vi "Run_6_of_6_Tests.vi"() -> ()   [LabVIEW 2019]
uses:
  <vilib>/Rock Robotics/WPI/ThirdParty/JAS_Junk/TrajLib/Trajectory_Library.lvlib
panel:
  out "Vector":bool
  out "Lead Lag":bool
  out "Pose3d":bool
  out "Transform3d":bool
  out "Rotation3d":bool
  out "Translation3d":bool
  out "Twist3d":bool
  out "Function Generator \nMatrix":bool
  out "LTV Unicycle \nController":bool
  out "LTV Diff Drive \nController":bool
  out "Time Interpolatable Rotation":bool
  out "Time Interpolatable Double":bool
  out "Time Interpolatable Boolean":bool
  out "Time Interpolatable Pose":bool
  out "Implicit Model Follower":bool
  out "Function Generator":bool
  out "Diff Drive Accel Limiter":bool
  out "String":string
  out "All Tests Finished":bool
  # "FORMAL TRAJECTORY / CONTROL LIBRARY TEST PROCEDURE"
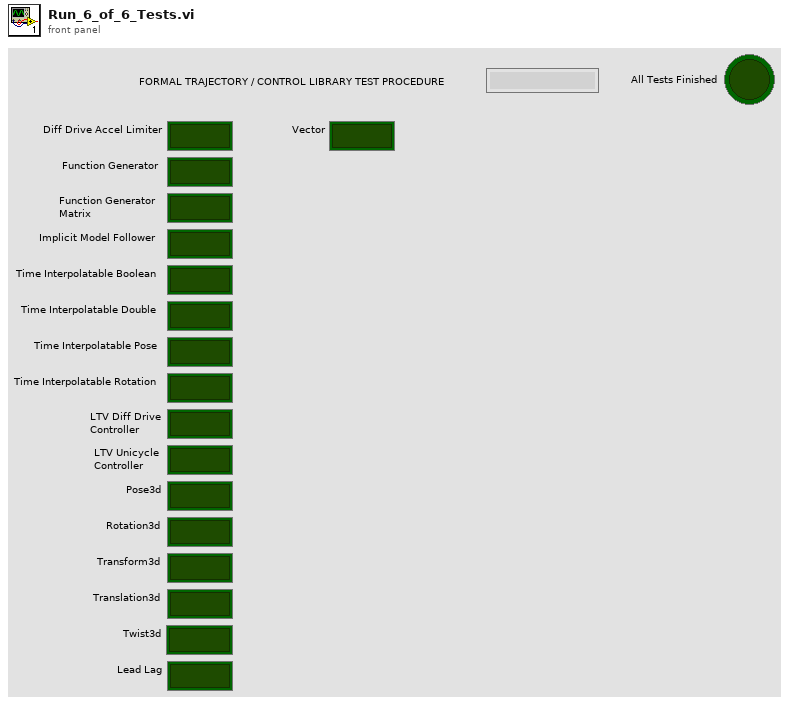
[diagram p1: front panel]
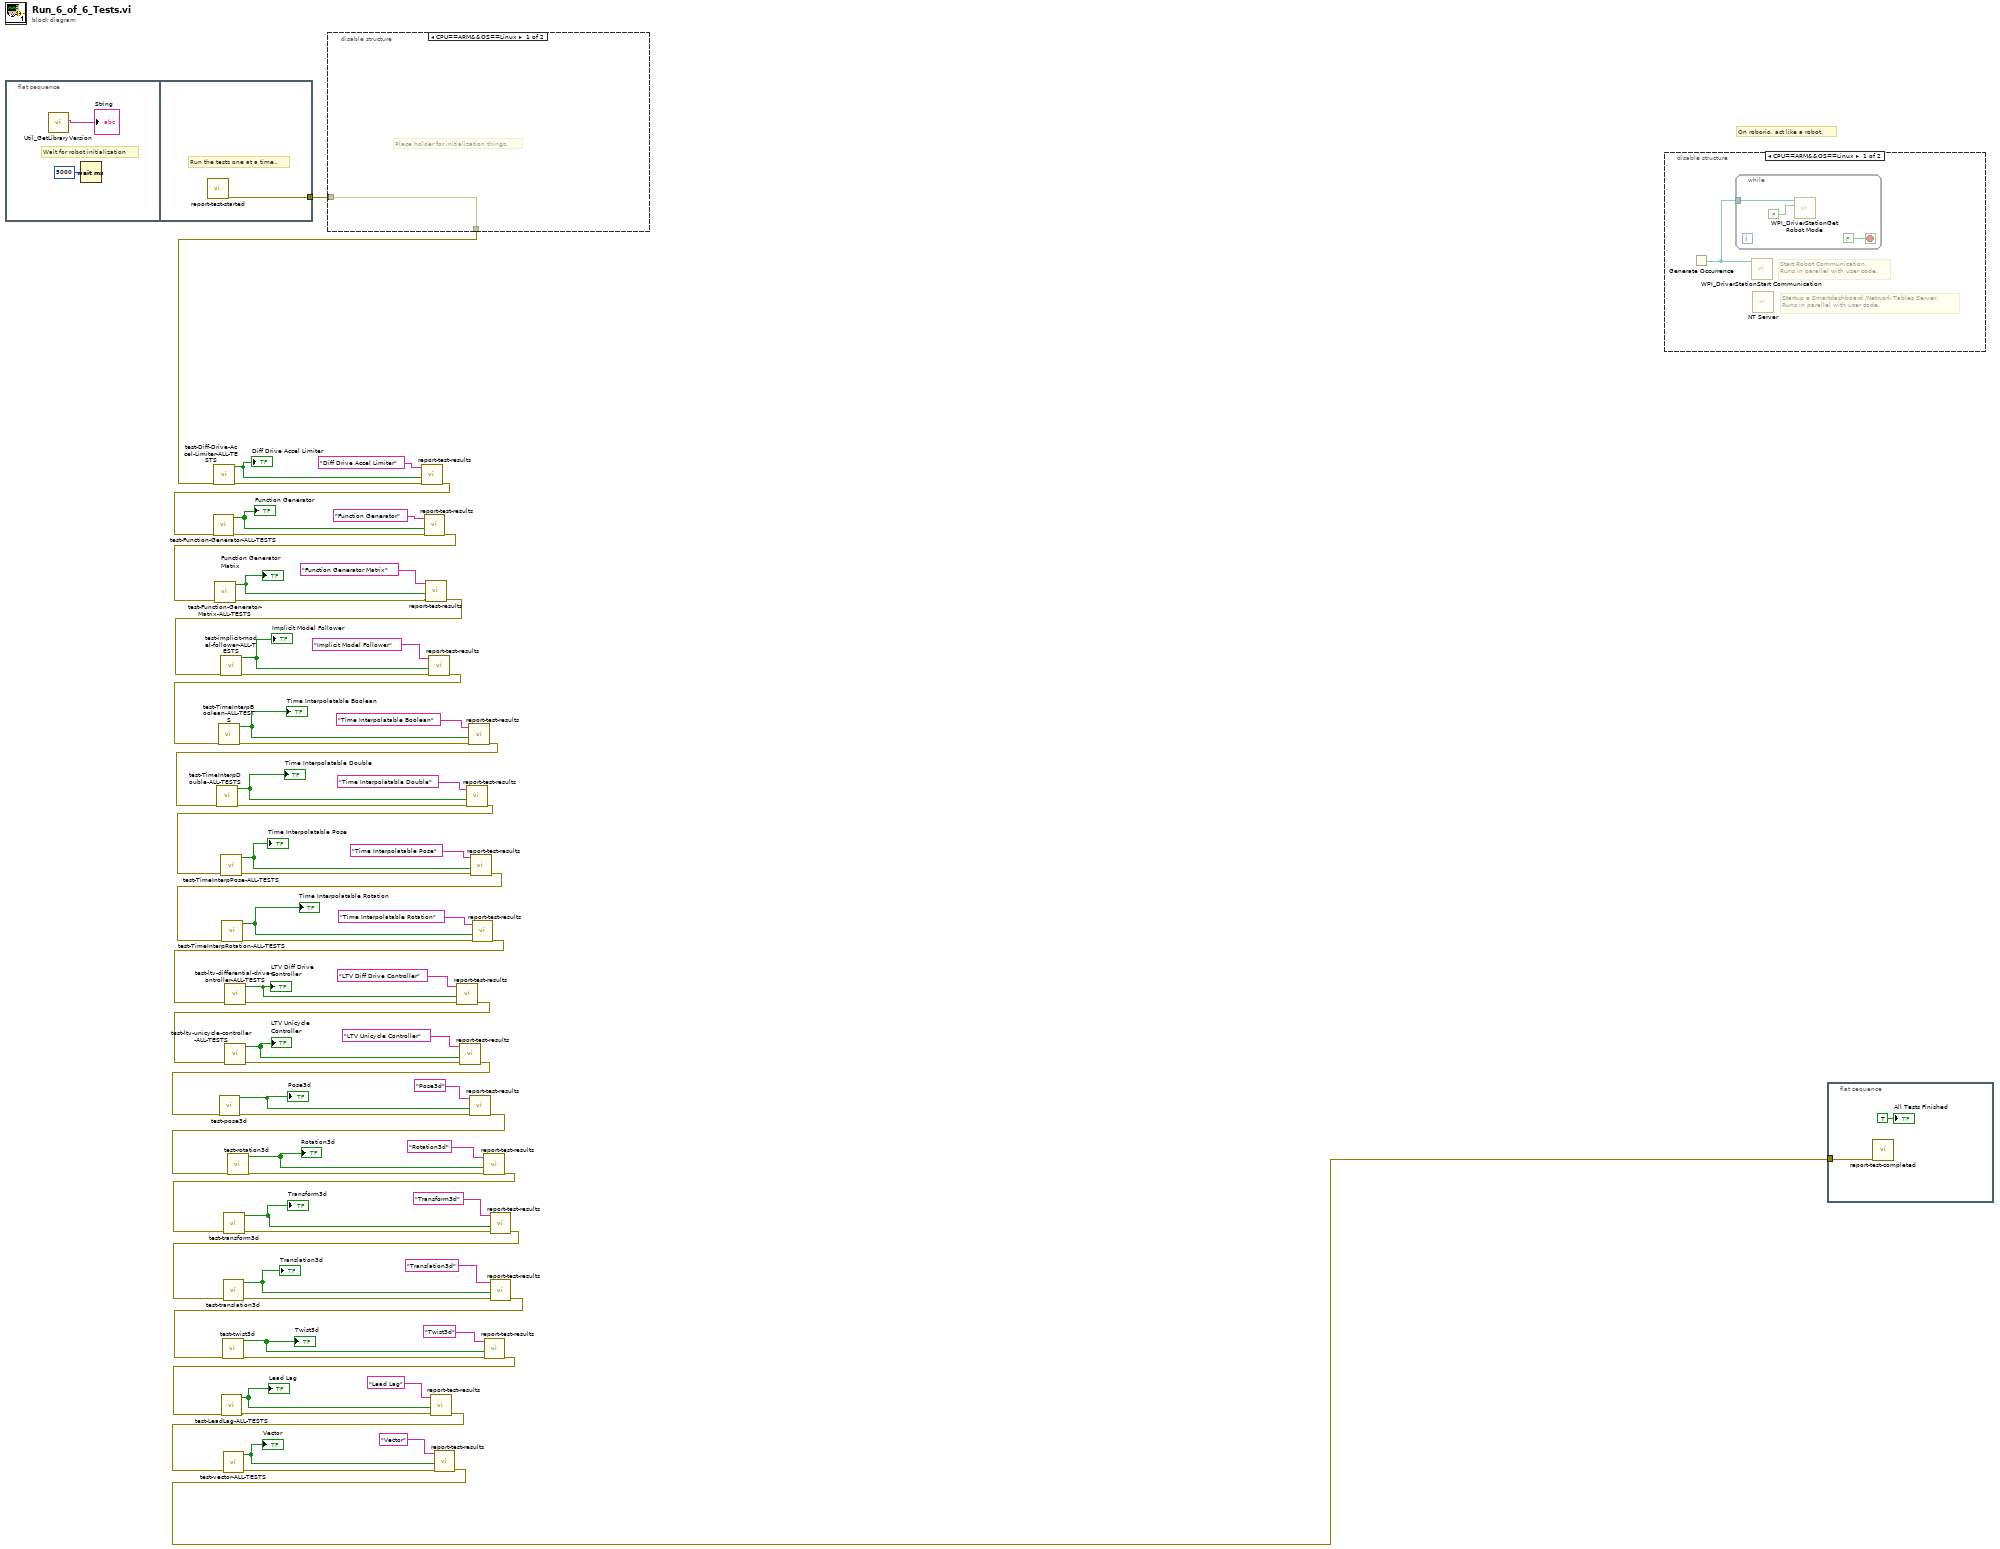
[diagram p0: block diagram]
diagram:
  # "On roborio, act like a robot."
  n1 = flat-sequence {
    tunnel: [w73] -> w70
    frame #0 {
      # "Wait for robot initialization"
      n2 = call <vilib>:"Util_GetLibraryVersion.vi"() -> ("TrajLibVersion"=→"String":string)  [unwired: 11 in]
      n3 = Wait (ms)(milliseconds to wait=u32 5000) -> ()  [unwired: 1 out]
    }
    frame #1 {
      # "Run the tests one at a time.."
      n4 = call "report-test-started.vi"() -> ("error out"=w73:errorcluster)  [unwired: 11 in]
    }
  }
  n5 = disable-structure shown="CPU==ARM&&OS==Linux" {
    disable-tunnel: w70 -> [w74 w75]
    disable-tunnel: [w74 w75] -> w66
    frame condition #0 {
      # "Place holder for initialization things."
    }
    frame condition #1 (active) {
    }
  }
  n6 = call "test-Diff-Drive-Accel-Limiter-ALL-TESTS.vi"("error in (no error)"=w66) -> ("error out"=w68:errorcluster, "All Passed"=w67:bool)  [unwired: 9 in]
  "Diff Drive Accel Limiter" <- w67
  n7 = call "report-test-results.vi"("error in (no error)"=w68, "TestPassed"=w67, "Test Name"="Diff Drive Accel Limiter") -> ("error out"=w62:errorcluster)  [unwired: 8 in]
  n8 = call "test-Function-Generator-ALL-TESTS.vi"("error in (no error)"=w62) -> ("error out"=w64:errorcluster, "All Passed"=w63:bool)  [unwired: 9 in]
  "Function Generator" <- w63
  n9 = call "report-test-results.vi"("error in (no error)"=w64, "TestPassed"=w63, "Test Name"="Function Generator") -> ("error out"=w32:errorcluster)  [unwired: 8 in]
  n10 = call "test-Function-Generator-Matrix-ALL-TESTS.vi"("error in (no error)"=w32) -> ("error out"=w34:errorcluster, "All Passed"=w33:bool)  [unwired: 9 in]
  "Function Generator \nMatrix" <- w33
  n11 = call "report-test-results.vi"("error in (no error)"=w34, "TestPassed"=w33, "Test Name"="Function Generator Matrix") -> ("error out"=w31:errorcluster)  [unwired: 8 in]
  n12 = call "test-implicit-model-follower-ALL-TESTS.vi"("error in (no error)"=w31) -> ("error out"=w60:errorcluster, "All Passed"=w59:bool)  [unwired: 9 in]
  "Implicit Model Follower" <- w59
  n13 = call "report-test-results.vi"("error in (no error)"=w60, "TestPassed"=w59, "Test Name"="Implicit Model Follower") -> ("error out"=w46:errorcluster)  [unwired: 8 in]
  n14 = call "test-TimeInterpBoolean-ALL-TESTS.vi"("error in (no error)"=w46) -> ("error out"=w54:errorcluster, "All Passed"=w51:bool)  [unwired: 9 in]
  "Time Interpolatable Boolean" <- w51
  n15 = call "report-test-results.vi"("error in (no error)"=w54, "TestPassed"=w51, "Test Name"="Time Interpolatable Boolean") -> ("error out"=w43:errorcluster)  [unwired: 8 in]
  n16 = call "test-TimeInterpDouble-ALL-TESTS.vi"("error in (no error)"=w43) -> ("error out"=w52:errorcluster, "All Passed"=w50:bool)  [unwired: 9 in]
  "Time Interpolatable Double" <- w50
  n17 = call "report-test-results.vi"("error in (no error)"=w52, "TestPassed"=w50, "Test Name"="Time Interpolatable Double") -> ("error out"=w44:errorcluster)  [unwired: 8 in]
  n18 = call "test-TimeInterpPose-ALL-TESTS.vi"("error in (no error)"=w44) -> ("error out"=w57:errorcluster, "All Passed"=w56:bool)  [unwired: 9 in]
  "Time Interpolatable Pose" <- w56
  n19 = call "report-test-results.vi"("error in (no error)"=w57, "TestPassed"=w56, "Test Name"="Time Interpolatable Pose") -> ("error out"=w45:errorcluster)  [unwired: 8 in]
  n20 = call "test-TimeInterpRotation-ALL-TESTS.vi"("error in (no error)"=w45) -> ("error out"=w48:errorcluster, "All Passed"=w47:bool)  [unwired: 9 in]
  "Time Interpolatable Rotation" <- w47
  n21 = call "report-test-results.vi"("error in (no error)"=w48, "TestPassed"=w47, "Test Name"="Time Interpolatable Rotation") -> ("error out"=w36:errorcluster)  [unwired: 8 in]
  n22 = call "test-ltv-differential-drive-controller-ALL-TESTS.vi"("error in (no error)"=w36) -> ("error out"=w39:errorcluster, "All Passed"=w40:bool)  [unwired: 9 in]
  "LTV Diff Drive \nController" <- w40
  n23 = call "report-test-results.vi"("error in (no error)"=w39, "TestPassed"=w40, "Test Name"="LTV Diff Drive Controller") -> ("error out"=w18:errorcluster)  [unwired: 8 in]
  n24 = call "test-ltv-unicycle-controller-ALL-TESTS.vi"("error in (no error)"=w18) -> ("error out"=w38:errorcluster, "All Passed"=w37:bool)  [unwired: 9 in]
  "LTV Unicycle \nController" <- w37
  n25 = call "report-test-results.vi"("error in (no error)"=w38, "TestPassed"=w37, "Test Name"="LTV Unicycle Controller") -> ("error out"=w11:errorcluster)  [unwired: 8 in]
  n26 = call "test-pose3d.vi"("error in (no error)"=w11) -> ("error out"=w13:errorcluster, "All PASSED"=w12:bool)  [unwired: 9 in]
  "Pose3d" <- w12
  n27 = call "report-test-results.vi"("error in (no error)"=w13, "TestPassed"=w12, "Test Name"="Pose3d") -> ("error out"=w10:errorcluster)  [unwired: 8 in]
  n28 = call "test-rotation3d.vi"("error in (no error)"=w10) -> ("error out"=w23:errorcluster, "ALL TESTS PASSED"=w22:bool)  [unwired: 9 in]
  "Rotation3d" <- w22
  n29 = call "report-test-results.vi"("error in (no error)"=w23, "TestPassed"=w22, "Test Name"="Rotation3d") -> ("error out"=w17:errorcluster)  [unwired: 8 in]
  n30 = call "test-transform3d.vi"("error in (no error)"=w17) -> ("error out"=w20:errorcluster, "All PASSED"=w19:bool)  [unwired: 9 in]
  "Transform3d" <- w19
  n31 = call "report-test-results.vi"("error in (no error)"=w20, "TestPassed"=w19, "Test Name"="Transform3d") -> ("error out"=w16:errorcluster)  [unwired: 8 in]
  n32 = call "test-translation3d.vi"("error in (no error)"=w16) -> ("error out"=w26:errorcluster, "All PASSED"=w25:bool)  [unwired: 9 in]
  "Translation3d" <- w25
  n33 = call "report-test-results.vi"("error in (no error)"=w26, "TestPassed"=w25, "Test Name"="Translation3d") -> ("error out"=w15:errorcluster)  [unwired: 8 in]
  n34 = call "test-twist3d.vi"("error in (no error)"=w15) -> ("error out"=w29:errorcluster, "All PASSED"=w28:bool)  [unwired: 9 in]
  "Twist3d" <- w28
  n35 = call "report-test-results.vi"("error in (no error)"=w29, "TestPassed"=w28, "Test Name"="Twist3d") -> ("error out"=w6:errorcluster)  [unwired: 8 in]
  n36 = call "test-LeadLag-ALL-TESTS.vi"("error in (no error)"=w6) -> ("error out"=w8:errorcluster, "All Passed"=w7:bool)  [unwired: 9 in]
  "Lead Lag" <- w7
  n37 = call "report-test-results.vi"("error in (no error)"=w8, "TestPassed"=w7, "Test Name"="Lead Lag") -> ("error out"=w2:errorcluster)  [unwired: 8 in]
  n38 = call "test-vector-ALL-TESTS.vi"("error in (no error)"=w2) -> ("error out"=w4:errorcluster, "All Passed"=w1:bool)  [unwired: 9 in]
  "Vector" <- w1
  n39 = call "report-test-results.vi"("error in (no error)"=w4, "TestPassed"=w1, "Test Name"="Vector") -> ("error out"=w3:errorcluster)  [unwired: 8 in]
  n40 = disable-structure shown="CPU==ARM&&OS==Linux" {
    frame condition #0 {
      # "Startup a Smartdashboard /Network Tables Server.\nRuns in parallel with user code."
      # "Start Robot Communication.\nRuns in parallel with user code."
      n41 = Generate Occurrence() -> (w76:refnum<k4>)
      n42 = while {
        tunnel: w76 -> [w79]
        stop <- FALSE stop-if-true
        n43 = call <vilib>:"WPI_DriverStationGet Robot Mode.vi"("Finish"=FALSE, "DS Occurrence"=w79) -> ()  [unwired: 10 out]
      }
      n44 = call <vilib>:"WPI_DriverStationStart Communication.vi"("occurrence"=w76) -> ()  [unwired: 2 in, 9 out]
      n45 = call <vilib>:"NT Server.vi"() -> ()  [unwired: 12 in]
    }
    frame condition #1 (active) {
    }
  }
  n46 = flat-sequence {
    tunnel: w3 -> [w80]
    frame #0 {
      n47 = call "report-test-completed.vi"("error in (no error)"=w80) -> ()  [unwired: 10 in, 1 out]
      "All Tests Finished" <- TRUE ("All Tests Finished")
    }
  }
